vi "ziModGetNodeValue.vi"   [LabVIEW 2009, in "Zurich Instruments LabOne.lvlib"]
doc: "This polymorphic vi sets values to <b>module</b> nodes specified by <b>Path</b> to <b>Value</b>."
uses:
  <instrlib>/Zurich Instruments LabOne/Zurich Instruments LabOne.lvlib
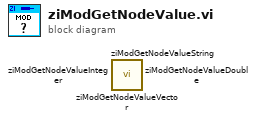
[diagram p0: block diagram]
diagram:
  n1 = call <instrlib>:"ziModGetNodeValueVector.vi"() -> ()  [unwired: 13 in, 3 out]
  n2 = call <instrlib>:"ziModGetNodeValueString.vi"() -> ()  [unwired: 13 in, 3 out]
  n3 = call <instrlib>:"ziModGetNodeValueInteger.vi"() -> ()  [unwired: 13 in, 3 out]
  n4 = call <instrlib>:"ziModGetNodeValueDouble.vi"() -> ()  [unwired: 13 in, 3 out]
